vi "4 memory dds 16SPC.vi"(0 "new PDW in":bool, 5 "free DDS before me?":bool, 7 "run":bool=TRUE, 9 "pdw in":T3 {"frequency shift" format="%#_12f"}, 11 "referenses":T1={"clock x2"="IO Socket\\Data Clock 2x", "Memory In"="pulse on memory", "Memory In 2"="pulse on memory", "Memory In 3"="pulse on memory", "Memory In 4"="pulse on memory"}) -> (4 "IQ out":T2[](array[typedef]), 6 "have free DDS":bool, 10 "state of every DDS":bool[](array[boolean]), 15 "output valid":bool)   [LabVIEW 2021]
doc: "transmit pulse with one free DDS inside.\nmust have no DDS before him (the distribute is to give the lowest mun DDS the pulse)"
uses:
  pulse_tx_vis/pdw.ctl
  pulse_tx_vis/CTL/mode_type.ctl
  <instrlib>/_niInstr/DSP/v1/Shared/Public/IQ Data.ctl
  <instrlib>/_niInstr/DSP/v1/Shared/niInstr DSP v1 Shared.lvlib
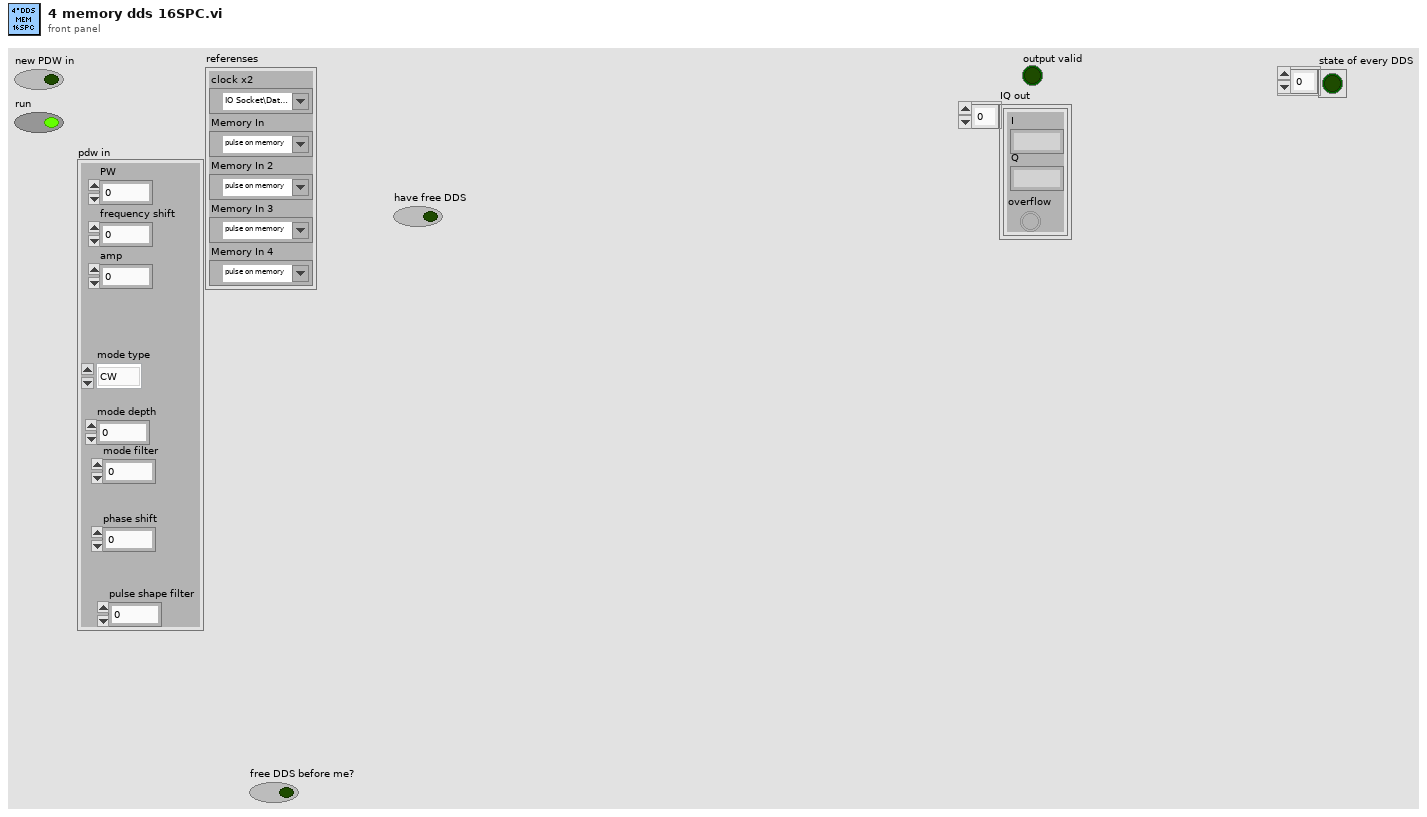
[diagram p1: front panel]
types:
  T1 = cluster{"clock x2":refnum<k21>, "Memory In":refnum<k21>, "Memory In 2":refnum<k21>, "Memory In 3":refnum<k21>, "Memory In 4":refnum<k21>}
  T2 = typedef "niInstr DSP v1 Shared.lvlib/IQ Data.ctl" = cluster{"I":fxp<+/-,18,1>, "Q":fxp<+/-,18,1>, "overflow":bool}
  T3 = typedef "pdw.ctl" = cluster{"PW":u32, "frequency shift":fxp<+/-,48,0>, "amp":fxp<+/-,18,1>, "mode type":T4, "mode depth":u32, "mode filter":u8, "phase shift":fxp<+/-,16,1>, "pulse shape filter":u8}
  T4 = typedef "mode_type.ctl" = enum8{"CW", "from memory 1", "NC - cw", "LFM", "BPSK", "QPSK"}
  T5 = cluster{"clock x2":refnum<k21>, "Memory In":refnum<k21>}
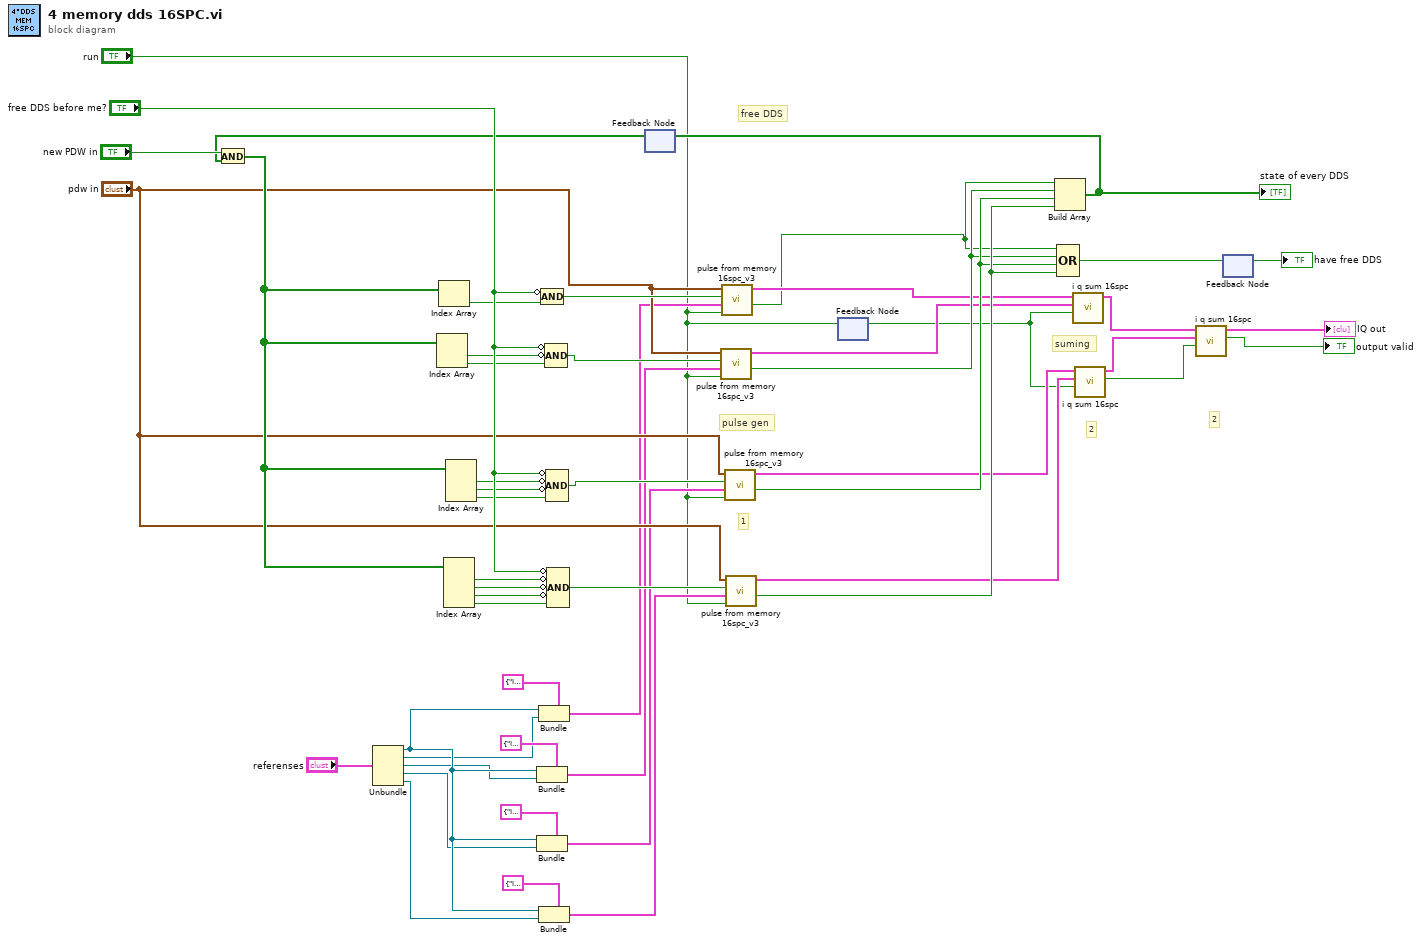
[diagram p0: block diagram]
diagram:
  # "1"
  # "2"
  # "2"
  # "free DDS"
  # "suming"
  # "pulse gen"
  n1 = Unbundle("referenses") -> ("clock x2"=w11:refnum<k21>, "Memory In"=w7:refnum<k21>, "Memory In 2"=w8:refnum<k21>, "Memory In 3"=w9:refnum<k21>, "Memory In 4"=w10:refnum<k21>)
  n2 = Bundle(cluster=T5 {"clock x2"="IO Socket\\Data Clock 2x", "Memory In"="pulse on memory"} ("referenses"), "clock x2"=w11, "Memory In"=w8) -> (w5:T5)
  n3 = Bundle(cluster=T5 {"clock x2"="IO Socket\\Data Clock 2x", "Memory In"="pulse on memory"} ("referenses"), "clock x2"=w11, "Memory In"=w9) -> (w4:T5)
  n4 = Bundle(cluster=T5 {"clock x2"="IO Socket\\Data Clock 2x", "Memory In"="pulse on memory"} ("referenses"), "clock x2"=w11, "Memory In"=w7) -> (w6:T5)
  n5 = Bundle(cluster=T5 {"clock x2"="IO Socket\\Data Clock 2x", "Memory In"="pulse on memory"} ("referenses"), "clock x2"=w11, "Memory In"=w10) -> (w3:T5)
  n6 = feedback #1() -> (w27:bool[])  [unwired: 1 in]
  n7 = And(x="new PDW in", y=w27) -> (x .and. y?=w26:bool[])
  n8 = Index Array(array=w26) -> (element #1=w38:bool, element #2=w36:bool)  [unwired: 2 in]
  n9 = Index Array(array=w26) -> (element=w34:bool)  [unwired: 1 in]
  n10 = Index Array(array=w26) -> (element #1=w46:bool, element #2=w45:bool, element #3=w44:bool, element #4=w43:bool)  [unwired: 4 in]
  n11 = Index Array(array=w26) -> (element #1=w42:bool, element #2=w41:bool, element #3=w40:bool)  [unwired: 3 in]
  n12 = Compound Arithmetic op=AND(invert "free DDS before me?", w34) -> (w35:bool)
  n13 = Compound Arithmetic op=AND(invert "free DDS before me?", invert w38, w36) -> (w37:bool)
  n14 = Compound Arithmetic op=AND(invert "free DDS before me?", invert w42, invert w41, w40) -> (w39:bool)
  n15 = Compound Arithmetic op=AND(invert "free DDS before me?", invert w46, invert w45, invert w44, w43) -> (w47:bool)
  n16 = call "pulse from memory 16spc_v3.vi"("run"="run", "referenses"=w5, "start this pulse"=w37, "PDW"="pdw in") -> ("free DDS"=w48:bool, "IQ_out"=w31:T2[])  [unwired: 5 in, 1 out]
  n17 = call "pulse from memory 16spc_v3.vi"("run"="run", "referenses"=w6, "start this pulse"=w35, "PDW"="pdw in") -> ("free DDS"=w17:bool, "IQ_out"=w30:T2[])  [unwired: 5 in, 1 out]
  n18 = call "pulse from memory 16spc_v3.vi"("run"="run", "referenses"=w4, "start this pulse"=w39, "PDW"="pdw in") -> ("free DDS"=w49:bool, "IQ_out"=w32:T2[])  [unwired: 5 in, 1 out]
  n19 = call "pulse from memory 16spc_v3.vi"("run"="run", "referenses"=w3, "start this pulse"=w47, "PDW"="pdw in") -> ("free DDS"=w50:bool, "IQ_out"=w33:T2[])  [unwired: 5 in, 1 out]
  n20 = feedback-in #2("run") -> ()
  n21 = feedback #2() -> (w1:bool)  [unwired: 1 in]
  n22 = Build Array(w17, w48, w49, w50) -> (w29:bool[])
  "state of every DDS" <- w29
  n23 = feedback-in #1(w29) -> ()
  n24 = Compound Arithmetic op=OR(w17, w48, w49, w50) -> (w25:bool)
  n25 = call "i q sum 16spc.vi"("input valid"=w1, "IQ in 2"=w31, "IQ in"=w30) -> ("IQ out"=w22:T2[])  [unwired: 7 in, 1 out]
  n26 = call "i q sum 16spc.vi"("input valid"=w1, "IQ in 2"=w33, "IQ in"=w32) -> ("output valid"=w20:bool, "IQ out"=w21:T2[])  [unwired: 7 in]
  n27 = call "i q sum 16spc.vi"("input valid"=w20, "IQ in 2"=w21, "IQ in"=w22) -> ("output valid"=→"output valid":bool, "IQ out"=→"IQ out":T2[])  [unwired: 7 in]
  n28 = feedback #3() -> (→"have free DDS":bool)  [unwired: 1 in]
  n29 = feedback-in #3(w25) -> ()
